vi "ConvertInputZUP.vi"(1 "Current":dbl) -> (0 "ZUP input voltage":dbl)   [LabVIEW 2012]
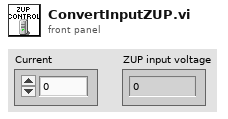
[diagram p1: front panel]
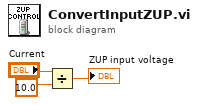
[diagram p0: block diagram]
diagram:
  n1 = Divide(x="Current", y=10.0) -> (x/y=→"ZUP input voltage":dbl)
